vi "Unevenly_spaced_spectra_ph.vi"(2 "Current Block No":i32, 3 "Shift in":dbl[](array[numeric]), 4 "U":dbl[](array[numeric]), 5 "Time":dbl[](array[numeric])) -> (0 "Sum E(F)":dbl[](array[numeric]), 1 "Freq":dbl[](array[numeric]))   [LabVIEW 2010]
uses:
  <vilib>/gmath/NI_Gmath.lvlib
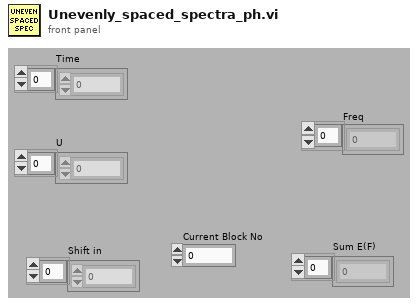
[diagram p1: front panel]
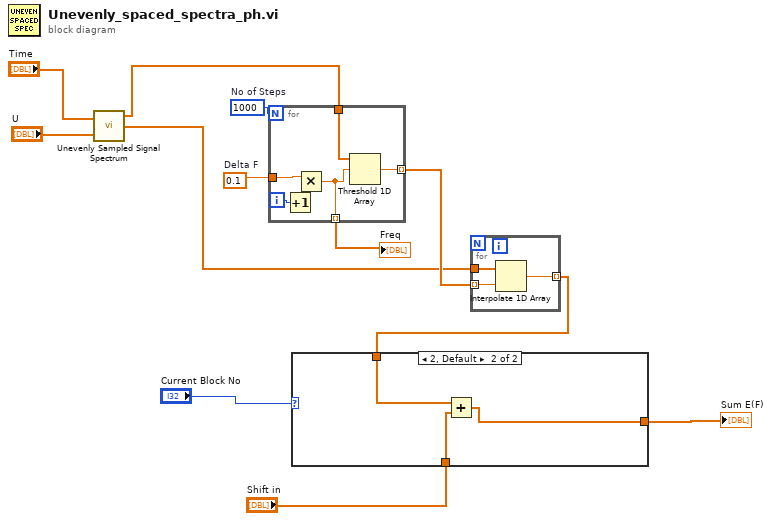
[diagram p0: block diagram]
diagram:
  w8 = 0.1  # Delta F
  w9 = 1000  # No of Steps
  n1 = call <vilib>:"Unevenly Sampled Signal Spectrum.vi"("XTime"="Time", "X"="U") -> ("Power Spectrum FFT {X} Frequency"=w7:dbl[], "Power Spectrum FFT {X}"=w6:dbl[])  [unwired: 1 out]
  n2 = for {
    N: w9 -> [_]
    tunnel: w8 -> [w17]
    tunnel: w7 -> [w16]
    tunnel: [w15] -> w10 mode=indexing
    tunnel: [w14] -> w1 mode=indexing
    i -> [w18]
    n3 = Increment(x=w18) -> (x+1=w13:i32)
    n4 = Multiply(x=w17, y=w13) -> (x*y=w14:dbl)
    n5 = Threshold 1D Array(2:w14, 3:w16) -> (0:w15:dbl)  [unwired: 1 out]
  }
  "Freq" <- w1
  n6 = for {
    tunnel: w6 -> [w21]
    tunnel: w10 -> [w20] mode=indexing
    tunnel: [w19] -> w4 mode=indexing
    n7 = Interpolate 1D Array(1:w20, 2:w21) -> (0:w19:dbl)
  }
  n8 = case shown="2, Default" "Current Block No" {
    tunnel: [w22 w23] -> w5
    tunnel: w4 -> [w22 w25]
    tunnel: "Shift in" -> [_ w24]
    frame 1 {
    }
    frame 2, Default {
      n9 = Add(x=w25, y=w24) -> (x+y=w23:dbl[])
    }
  }
  "Sum E(F)" <- w5
